vi "Get Topmost Block Diagram.vi"(8 "error in (no error)":errorcluster, 11 "Application reference":refnum<vi>) -> (0 "error out":errorcluster, 2 "Reference to Diagram":refnum<vi>, 3 "Vi refence for top most block diagram":refnum<vi>)   [LabVIEW 2012, in "Scripting Tools.lvlib"]
doc: "Get a reference to the Vi and block diagram of the Vi whose block diagram window is topmost"
uses:
  <userlib>/_LAVAcr/Scripting Tools/Scripting Tools.lvlib
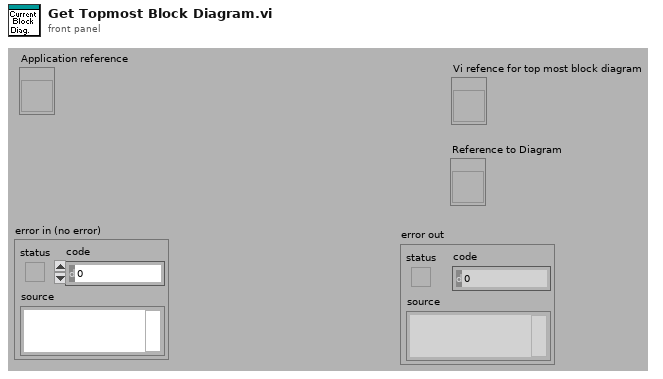
[diagram p1: front panel]
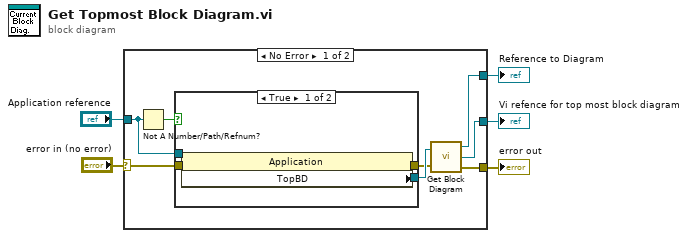
[diagram p0: block diagram]
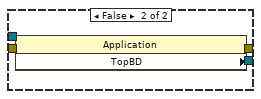
[diagram p2: hidden frame]
diagram:
  n1 = case shown="No Error" "error in (no error)" {
    selector: "error in (no error)" -> [w9 w21]
    tunnel: [w12 _] -> w5
    tunnel: [w11 _] -> w4
    tunnel: [w10 w21] -> w3
    tunnel: "Application reference" -> [w8 _]
    frame No Error {
      n2 = Not A Number/Path/Refnum?(number/path/refnum=w8) -> (NaN/Path/Refnum?=w7:bool)
      n3 = case shown="True" w7 {
        tunnel: [w16 w20] -> w13
        tunnel: w9 -> [w15 w19]
        tunnel: w8 -> [_ w18]
        tunnel: [w14 w17] -> w6
        frame True {
          n4 = property class="Application"(error in=w15) -> (error out=w14:errorcluster, "TopBD"=w16:refnum<vi>)  [unwired: 1 in, 1 out]
        }
        frame False {
          n5 = property class="Application"(reference=w18, error in=w19) -> (error out=w17:errorcluster, "TopBD"=w20:refnum<vi>)  [unwired: 1 out]
        }
      }
      n6 = call "Get Block Diagram.vi"("vi refnum in"=w13, "error in (no error)"=w6) -> ("Diagram"=w11:refnum<vi>, "vi refnum out"=w12:refnum<vi>, "error out"=w10:errorcluster)
    }
    frame Error {
    }
  }
  "error out" <- w3
  "Vi refence for top most block diagram" <- w5
  "Reference to Diagram" <- w4
